vi "Is Red Pitaya.vi"(7 "Acceptable logic tags":u16[](array[numeric])=[101, 102], 8 "Error In":errorcluster, 10 "Timeout":i32=100, 11 "Server address":string="192.168.1.100") -> (0 "Error Out":errorcluster, 2 "IDN response":u32=1 format="0x%x (%d)", 3 "Red Pitaya":bool, 4 "Error cleared?":bool, 5 "Logic tag out":u16)   [LabVIEW 2016, in "RP Communicator.lvclass"]
uses:
  RP Communicator.lvclass
  RP Communicator.lvclass/RP Communicator.ctl
  Write Timeout.vi
  <vilib>/Utility/error.llb/Error Cluster From Error Code.vi
  <vilib>/ErrorRing/Error Ring.xnode
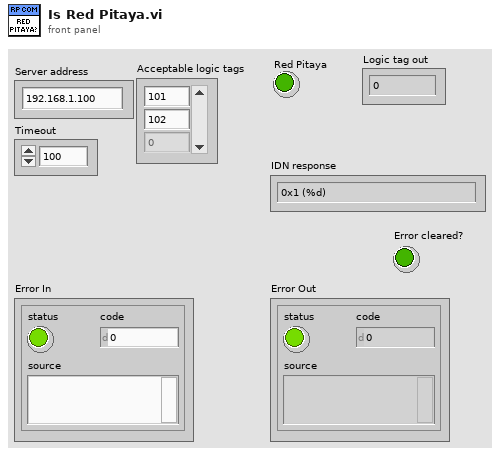
[diagram p1: front panel]
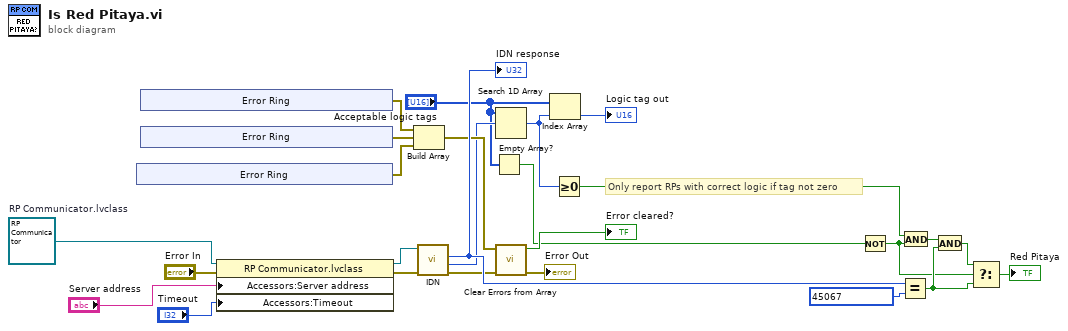
[diagram p0: block diagram]
diagram:
  w26 = refnum<class "RP Communicator.lvclass"> refnum  # RP Communicator.lvclass
  # "Only report RPs with correct logic if tag not zero"
  n1 = xnode "Error Ring"() -> ("error out"=w11:errorcluster)
  n2 = xnode "Error Ring"() -> ("error out"=w10:errorcluster)
  n3 = xnode "Error Ring"() -> ("error out"=w12:errorcluster)
  n4 = property class="RP Communicator.lvclass"(reference=w26, error in="Error In", "Accessors:Server address"="Server address", "Accessors:Timeout"="Timeout") -> (reference out=w23:refnum<class "RP Communicator.lvclass">, error out=w22:errorcluster)
  n5 = Build Array(w10, w12, w11) -> (w9:errorcluster[])
  n6 = call-dynamic "IDN.vi"("error in (no error)"=w22, "RP Communicator in"=w23) -> ("error out"=w14:errorcluster, "Logic tag"=w7:u16, "IDN response"=w18:u32)  [unwired: 6 in, 1 out]
  "IDN response" <- w18
  n7 = Empty Array?(array="Acceptable logic tags") -> (empty?=w4:bool)
  n8 = Search 1D Array(1D array="Acceptable logic tags", element=w7) -> (index of element=w2:i32)  [unwired: 1 in]
  n9 = call "Clear Errors from Array.vi"("Error In"=w14, "Errors to clear"=w9) -> ("Error Out"=→"Error Out":errorcluster, "specific error cleared?"=→"Error cleared?":bool)  [unwired: 8 in]
  n10 = Index Array(array="Acceptable logic tags", index=w2) -> (element=→"Logic tag out":u16)
  n11 = Greater Or Equal To 0?(x=w2) -> (x >= 0?=w1:bool)
  n12 = Not(x=w4) -> (.not. x?=w3:bool)
  n13 = Equal?(x=w18, y=u32 45067 ("IDN response")) -> (x = y?=w16:bool)
  n14 = And(x=w1, y=w3) -> (x .and. y?=w15:bool)
  n15 = And(x=w15, y=w16) -> (x .and. y?=w17:bool)
  n16 = Select(t=w17, s=w3, f=w16) -> (s? t:f=→"Red Pitaya":bool)
